vi "Configure.vi"(8 "error in (no error)":errorcluster, 11 "GRMActor in":refnum<class "LaserController.lvclass">) -> (0 "error out":errorcluster, 3 "GRMActor out":refnum<class "LaserController.lvclass">)   [LabVIEW 2020, in "LaserController.lvlib" / "LaserController.lvclass"]
uses:
  LaserController.lvclass
  Model/Hardware Abstraction Layer/Component/GenericActor/GenericActor/GenericController.lvclass
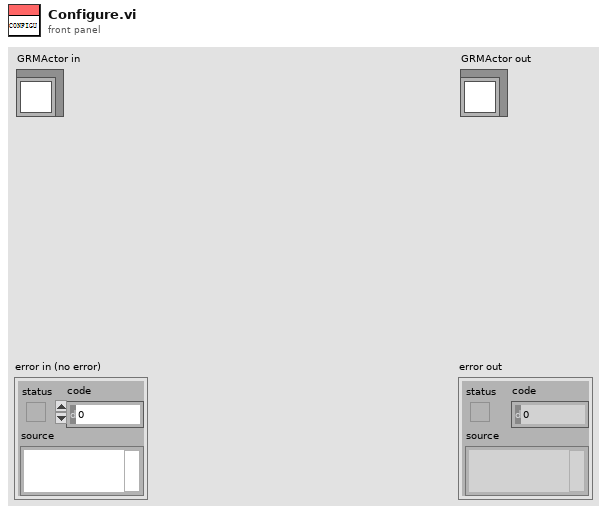
[diagram p1: front panel]
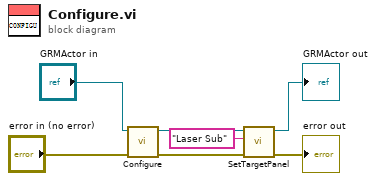
[diagram p0: block diagram]
diagram:
  n1 = call-parent "Configure.vi"("error in (no error)"="error in (no error)", "GRMActor in"="GRMActor in") -> ("error out"=w7:errorcluster, "GRMActor out"=w3:refnum<class "LaserController.lvclass">)  [unwired: 8 in]
  n2 = call-dynamic "SetTargetPanel.vi"("error in (no error)"=w7, "TargetPanel"="Laser Sub", "GRMActor in"=w3) -> ("error out"=→"error out":errorcluster, "GRMActor out"=→"GRMActor out":refnum<class "LaserController.lvclass">)  [unwired: 7 in]
